vi "Read TCP Data.vi"(7 "bytes to read":i32, 8 "error in":errorcluster, 9 "timeout ms (25000)":i32, 10 "mode (standard)":T1(ring), 11 "Module ID":i32=-1) -> (0 "error out":errorcluster)   [LabVIEW 2018, in "TCP-IP Engine.lvlib"]
doc: "This Request Event will request the TCP-IP Module to read the data from the respective connection.\n_____\nCreated using DQMH Event Scripter 7.0.1.1316."
uses:
  TCP-IP Engine.lvlib
  Read TCP Data Argument--cluster.ctl
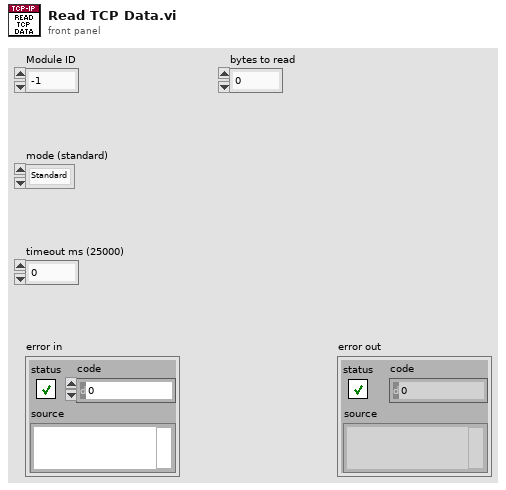
[diagram p1: front panel]
types:
  T1 = enum16{"Standard", "Buffered", "CRLF", "Immediate"}
  T2 = typedef "TCP-IP Engine.lvlib/Read TCP Data Argument--cluster.ctl" = cluster{"Module ID":i32, "mode (standard)":enum16{"Standard", "Buffered", "CRLF", "Immediate"}, "timeout ms (25000)":i32, "bytes to read":i32}
  T3 = typedef "TCP-IP Engine.lvlib/Request Events--cluster.ctl" = cluster{"Stop Module":refnum<user-event>, "Show Panel":refnum<user-event>, "Hide Panel":refnum<user-event>, "Show Diagram":refnum<user-event>, "Get Module Execution Status":refnum<user-event>, "TCP-Open Connection":refnum<user-event>, "Read TCP Data":refnum<user-event>, "TCP-Write":refnum<user-event>, "TCP-Close Connection":refnum<user-event>}
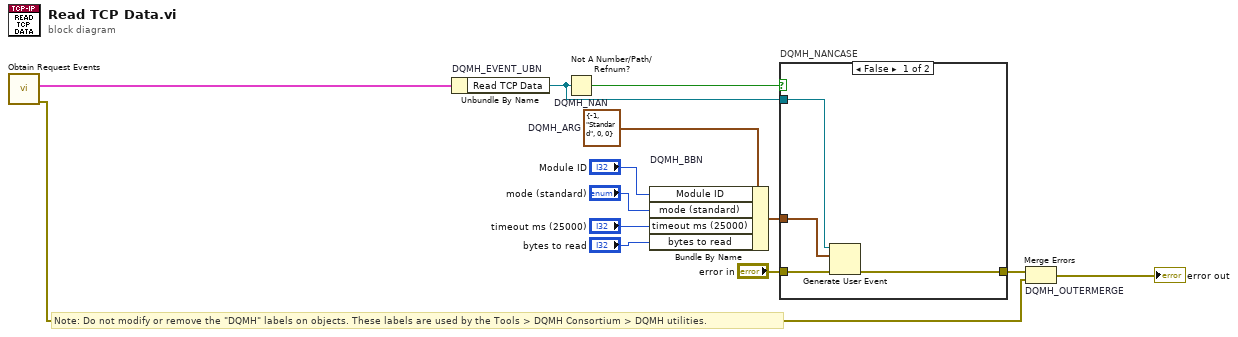
[diagram p0: block diagram]
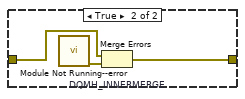
[diagram p2: hidden frame]
diagram:
  w7 = T2 {"Module ID"=-1, "mode (standard)"=enum."Standard", "timeout ms (25000)"=0, "bytes to read"=0}  # DQMH_ARG
  # "Note: Do not modify or remove the \"DQMH\" labels on objects. These labels are used by the Tools > DQMH Consortium > DQMH utilities."
  n1 = call "Obtain Request Events.vi"() -> ("error out"=w2:errorcluster, "TCP-IP Engine Request Events"=w1:T3)  [unwired: 10 in]
  n2 = Unbundle By Name "DQMH_EVENT_UBN"(w1) -> ("Read TCP Data"=w9:refnum<user-event>)
  n3 = Not A Number/Path/Refnum? "DQMH_NAN"(number/path/refnum=w9) -> (NaN/Path/Refnum?=w10:bool)
  n4 = Bundle By Name "DQMH_BBN"(cluster=w7, "Module ID"="Module ID", "mode (standard)"="mode (standard)", "timeout ms (25000)"="timeout ms (25000)", "bytes to read"="bytes to read") -> (w11:T2)
  n5 = case "DQMH_NANCASE" shown="False" w10 {
    tunnel: "error in" -> [w17 w20]
    tunnel: [w16 w19] -> w8
    tunnel: w9 -> [w15 _]
    tunnel: w11 -> [w14 _]
    frame False {
      n6 = Generate User Event(user event=w15, event data cluster=w14, error in=w17) -> (error out=w16:errorcluster)  [unwired: 1 in, 1 out]
    }
    frame True {
      n7 = call "Module Not Running--error.vi"() -> ("error out"=w18:errorcluster)  [unwired: 11 in]
      n8 = Merge Errors "DQMH_INNERMERGE"(w20, w18) -> (w19:errorcluster)
    }
  }
  n9 = Merge Errors "DQMH_OUTERMERGE"(w8, w2) -> (→"error out":errorcluster)
